vi "Vision4.vi"   [LabVIEW 2016]
uses:
  Robot Global Data.vi
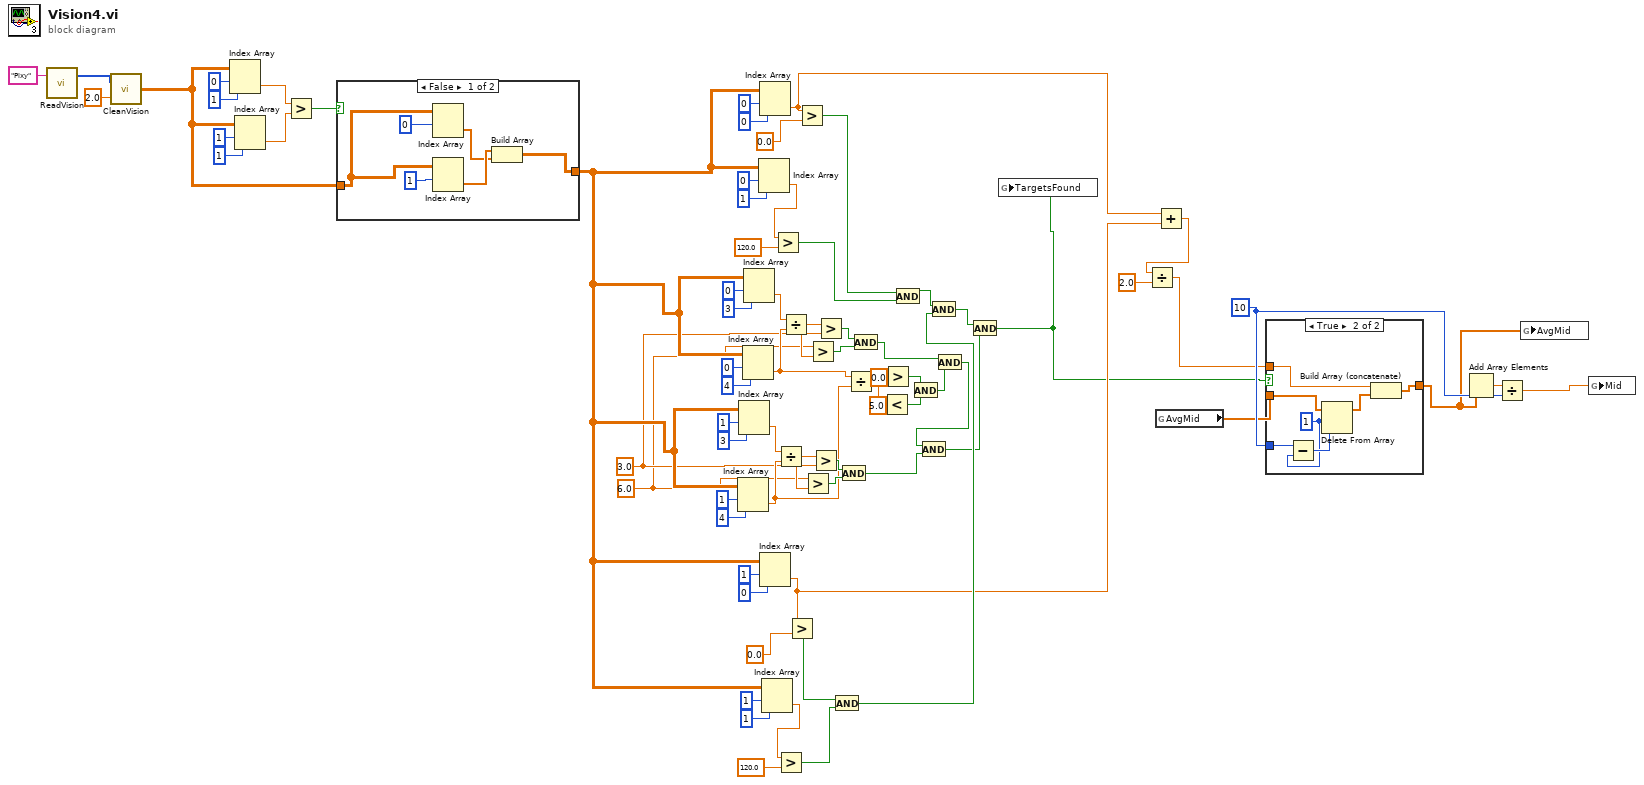
[diagram p0: block diagram]
diagram:
  w9 = 6.0 ("x")
  w10 = 3.0 ("y")
  w64 = 10
  n1 = call "ReadVision.vi"("Name"="Pixy") -> ("Target Data"=w4:u16[])  [unwired: 2 in]
  n2 = call "CleanVision.vi"("Targets"=2.0, "Input"=w4) -> ("Output"=w2:dbl[][])
  n3 = Index Array(array=w2, index (row)=0, index (col)=1 ("disabled index (col)")) -> (element=w13:dbl)
  n4 = Index Array(array=w2, index (row)=1, index (col)=1 ("disabled index (col)")) -> (element=w14:dbl)
  n5 = Greater?(x=w13, y=w14) -> (0:w12:bool)
  n6 = case shown="False" w12 {
    tunnel: w2 -> [w79 w81]
    tunnel: [w75 w81] -> w11
    frame False {
      n7 = Index Array(array=w79, index (row)=0) -> (element=w76:dbl[])  [unwired: 1 in]
      n8 = Index Array(array=w79, index (row)=1) -> (element=w77:dbl[])  [unwired: 1 in]
      n9 = Build Array(w77, w76) -> (w75:dbl[][])
    }
    frame True {
    }
  }
  n10 = Index Array(array=w11, index (row)=1, index (col)=4 ("disabled index (col)")) -> (element=w35:dbl)
  n11 = Index Array(array=w11, index (row)=1, index (col)=3 ("disabled index (col)")) -> (element=w40:dbl)
  n12 = Index Array(array=w11, index (row)=0, index (col)=4 ("disabled index (col)")) -> (element=w36:dbl)
  n13 = Index Array(array=w11, index (row)=0, index (col)=3 ("disabled index (col)")) -> (element=w48:dbl)
  n14 = Index Array(array=w11, index (row)=0, index (col)=1 ("disabled index (col)")) -> (element=w68:dbl)
  n15 = Index Array(array=w11, index (row)=0, index (col)=0 ("disabled index (col)")) -> (element=w20:dbl)
  n16 = Index Array(array=w11, index (row)=1, index (col)=0 ("disabled index (col)")) -> (element=w19:dbl)
  n17 = Index Array(array=w11, index (row)=1, index (col)=1 ("disabled index (col)")) -> (element=w58:dbl)
  n18 = Greater?(x=w68, y=120.0) -> (0:w65:bool)
  n19 = Divide(x=w40, y=w35) -> (x/y=w39:dbl)
  n20 = Greater?(x=w58, y=120.0) -> (0:w55:bool)
  n21 = Divide(x=w48, y=w36) -> (x/y=w47:dbl)
  n22 = Greater?(x=w19, y=0.0) -> (0:w56:bool)
  n23 = Greater?(x=w20, y=0.0) -> (0:w66:bool)
  n24 = Greater?(x=w9, y=w39) -> (0:w37:bool)
  n25 = Greater?(x=w9, y=w47) -> (0:w46:bool)
  n26 = Greater?(x=w39, y=w10) -> (0:w38:bool)
  n27 = Greater?(x=w47, y=w10) -> (0:w45:bool)
  n28 = And(x=w56, y=w55) -> (x .and. y?=w53:bool)
  n29 = And(x=w38, y=w37) -> (x .and. y?=w27:bool)
  n30 = Divide(x=w36, y=w35) -> (x/y=w32:dbl)
  n31 = And(x=w45, y=w46) -> (x .and. y?=w29:bool)
  n32 = Less?(x=w32, y=5.0) -> (x < y?=w30:bool)
  n33 = Greater?(x=w32, y=0.0) -> (0:w31:bool)
  n34 = And(x=w66, y=w65) -> (x .and. y?=w54:bool)
  n35 = And(x=w31, y=w30) -> (x .and. y?=w28:bool)
  n36 = And(x=w54, y=w53) -> (x .and. y?=w24:bool)
  n37 = And(x=w29, y=w28) -> (x .and. y?=w26:bool)
  n38 = And(x=w26, y=w27) -> (x .and. y?=w25:bool)
  n39 = And(x=w24, y=w25) -> (x .and. y?=w8:bool)
  n40 = global write "Robot Global Data.vi" "TargetsFound"(w8) -> ()
  n41 = Add(x=w20, y=w19) -> (x+y=w23:dbl)
  n42 = Divide(x=w23, y=2.0) -> (x/y=w22:dbl)
  n43 = global read "Robot Global Data.vi" "AvgMid"() -> (w1:dbl[])
  n44 = case shown="True" w8 {
    tunnel: w22 -> [_ w89]
    tunnel: [w82 w88] -> w7
    tunnel: w1 -> [w82 w86]
    tunnel: w64 -> [_ w83]
    frame False {
    }
    frame True {
      w84 = 1 ("length")
      n45 = Subtract(x=w83, y=w84) -> (x-y=w85:i32)
      n46 = Delete From Array(array=w86, length=w84, index=w85) -> (array with subset deleted=w87:dbl[])  [unwired: 1 out]
      n47 = Build Array (concatenate)(w89, w87) -> (w88:dbl[])
    }
  }
  n48 = Add Array Elements(numeric array=w7) -> (sum=w72:dbl)
  n49 = Divide(x=w72, y=w64) -> (x/y=w6:dbl)
  n50 = global write "Robot Global Data.vi" "AvgMid"(w7) -> ()
  n51 = global write "Robot Global Data.vi" "Mid"(w6) -> ()
